vi "USRP Convert Tx Config.vi"(0 "tx config":T3={"rf enable 0"=FALSE, "rf config 0"={"antenna"="TX1", "frequency"=2000000000.0, "lo frequency"=-1.0, "level"=0.0}, "rf enable 1"=FALSE, "rf config 1"={"antenna"="TX1", "frequency"=2000000000.0, "lo frequency"=-1.0, "level"=0.0}, "transfer mode"=enum."Finite", "sample rate"=10000000.0, "number of samples"=8192, "start trigger"=enum."Immediate", "tone frequency"=100000.0} {"tone frequency" format="%#.3pHz"; "sample rate" format="%#.3pS/s"; "rf config 0"."level" format="%#_gdBm"; "rf config 0"."lo frequency" format="%#.3pHz"; "rf config 0"."frequency" format="%#.3pHz"; "rf config 1"."level" format="%#_gdBm"; "rf config 1"."lo frequency" format="%#.3pHz"; "rf config 1"."frequency" format="%#.3pHz"}) -> (4 "tx config out":T2={"channel configuration"=[], "transfer mode"=enum."Finite", "sample rate"=10000000.0, "number of samples"=8192, "start trigger"=enum."Immediate", "tone frequency"=100000.0} {"channel configuration"."channel configuration"."frequency" format="%#.3pHz"; "channel configuration"."channel configuration"."lo frequency" format="%#.3pHz"; "channel configuration"."channel configuration"."level" format="%#_gdBm"; "tone frequency" format="%#.3pHz"; "sample rate" format="%#.3pS/s"})   [LabVIEW 2016]
uses:
  USRP Start Trigger.ctl
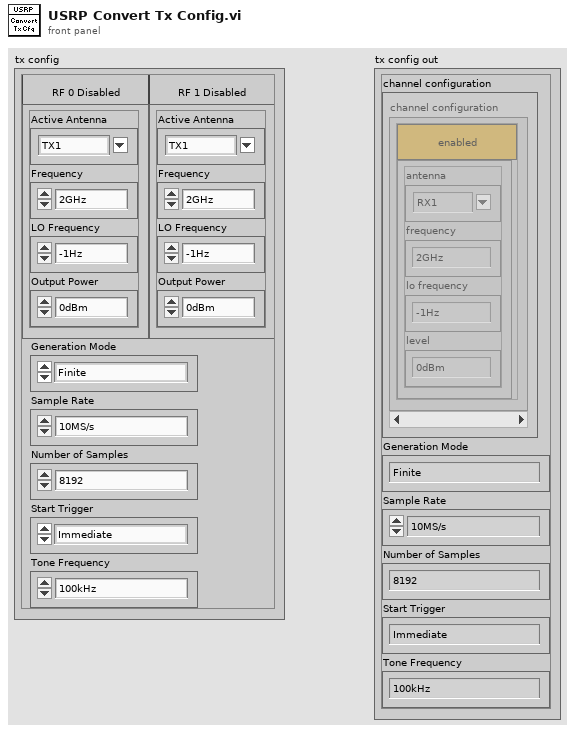
[diagram p1: front panel]
types:
  T1 = typedef "USRP Start Trigger.ctl" = enum8{"Software", "Digital Edge", "Rx Start Trigger", "Tx Start Trigger", "Immediate", "Future Time Event"}
  T2 = cluster{"channel configuration":cluster{"channel enable":bool, "channel configuration":cluster{"antenna":string, "frequency":dbl, "lo frequency":dbl, "level":dbl}}[], "transfer mode":enum16{"Finite", "Continuous"}, "sample rate":dbl, "number of samples":u32, "start trigger":T1, "tone frequency":dbl}
  T3 = cluster{"rf enable 0":bool, "rf config 0":cluster{"antenna":string, "frequency":dbl, "lo frequency":dbl, "level":dbl}, "rf enable 1":bool, "rf config 1":cluster{"antenna":string, "frequency":dbl, "lo frequency":dbl, "level":dbl}, "transfer mode":enum16{"Finite", "Continuous"}, "sample rate":dbl, "number of samples":u32, "start trigger":T1, "tone frequency":dbl}
  T4 = cluster{"antenna":string, "frequency":dbl, "lo frequency":dbl, "level":dbl}
  T5 = cluster{"rf enable 0":bool, "rf config 0":cluster{"antenna":string, "frequency":dbl, "lo frequency":dbl, "level":dbl}}
  T6 = cluster{"rf enable 1":bool, "rf config 1":cluster{"antenna":string, "frequency":dbl, "lo frequency":dbl, "level":dbl}}
  T7 = cluster{"rf enable 1":bool, "rf config 1":cluster{"antenna":string, "frequency":dbl, "lo frequency":dbl, "level":dbl}}[]
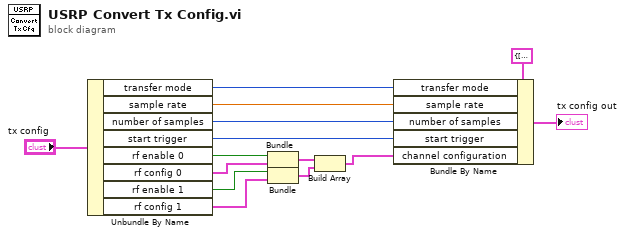
[diagram p0: block diagram]
diagram:
  n1 = Unbundle By Name("tx config") -> ("transfer mode"=w13:enum16{"Finite", "Continuous"}, "sample rate"=w12:dbl, "number of samples"=w11:u32, "start trigger"=w10:T1, "rf enable 0"=w7:bool, "rf config 0"=w6:T4, "rf enable 1"=w5:bool, "rf config 1"=w4:T4)
  n2 = Bundle("rf enable 0"=w7, "rf config 0"=w6) -> (w9:T5)  [unwired: 1 in]
  n3 = Bundle("rf enable 1"=w5, "rf config 1"=w4) -> (w8:T6)  [unwired: 1 in]
  n4 = Build Array(w9, w8) -> (w3:T7)
  n5 = Bundle By Name(cluster=T2 {"channel configuration"=[], "transfer mode"=enum."Finite", "sample rate"=10000000.0, "number of samples"=8192, "start trigger"=enum."Immediate", "tone frequency"=100000.0} ("tx config"), "transfer mode"=w13, "sample rate"=w12, "number of samples"=w11, "start trigger"=w10, "channel configuration"=w3) -> (→"tx config out":T2)
